vi "ExSubCloseExperiment.vi"(1 "error in (no error)":errorcluster, 2 "Handles In":T1) -> (0 "error out":errorcluster)   [LabVIEW 2010]
panel:
  # "ExSubCloseExperiment:\nThis Sub VI closes an experiment."
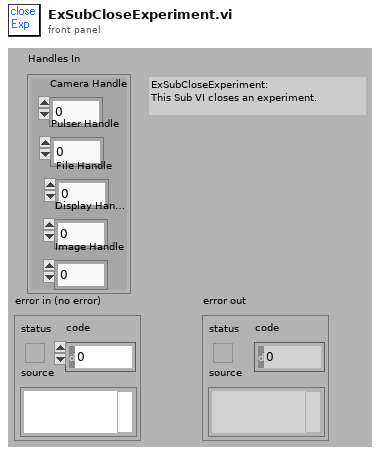
[diagram p1: front panel]
types:
  T1 = cluster{"Camera Handle":u32, "Pulser Handle":u32, "File Handle":u32, "Display Handle":u32, "Image Handle":u32}
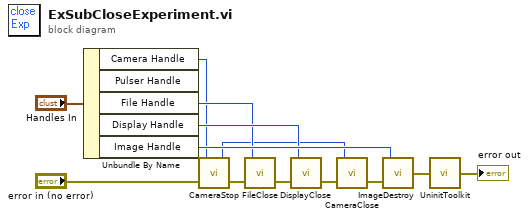
[diagram p0: block diagram]
diagram:
  n1 = Unbundle By Name("Handles In") -> ("Camera Handle"=w1:u32, "File Handle"=w9:u32, "Display Handle"=w10:u32, "Image Handle"=w11:u32)  [unwired: 1 out]
  n2 = call <userlib>:"CameraStop.vi"("error in"="error in (no error)", "Camera Handle"=w1) -> ("error out"=w6:errorcluster, "Camera Handle"=w7:u32)
  n3 = call <userlib>:"FileClose.vi"("error in"=w6, "File Handle"=w9) -> ("error out"=w12:errorcluster)
  n4 = call <userlib>:"DisplayClose.vi"("error in"=w12, "Display Handle"=w10) -> ("error out"=w4:errorcluster)
  n5 = call <userlib>:"CameraClose.vi"("error in"=w4, "Camera Handle"=w7) -> ("error out"=w3:errorcluster)
  n6 = call <userlib>:"ImageDestroy.vi"("error in"=w3, "Data handle"=w11) -> ("error out"=w2:errorcluster)
  n7 = call <userlib>:"UninitToolkit.vi"("error in"=w2) -> ("error out"=→"error out":errorcluster)
